vi "Data2Array.vi"(1 "ArrayLen":dbl, 2 "date":dbl) -> (0 "Array":dbl[](array[numeric]))   [LabVIEW 2014, in "Xgraph.xctl"]
uses:
  Xgraph.xctl
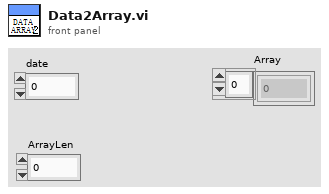
[diagram p1: front panel]
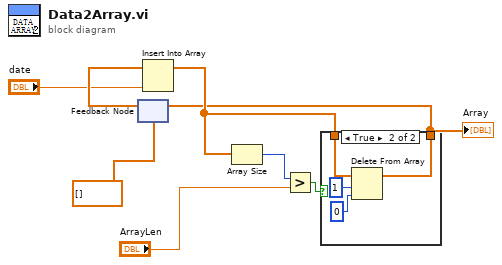
[diagram p0: block diagram]
diagram:
  n1 = feedback #1(dbl[] []) -> (w8:dbl[])
  n2 = Insert Into Array(array=w8, new element="date") -> (w4:dbl[])  [unwired: 1 in]
  n3 = Array Size(array=w4) -> (size(s)=w6:i32)
  n4 = Greater?(x=w6, y="ArrayLen") -> (0:w5:bool)
  n5 = case shown="True" w5 {
    tunnel: w4 -> [w9 w13]
    tunnel: [w9 w12] -> w2
    frame False {
    }
    frame True {
      n6 = Delete From Array(array=w13, length=1, index=0) -> (array with subset deleted=w12:dbl[])  [unwired: 1 out]
    }
  }
  "Array" <- w2
  n7 = feedback-in #1(w2) -> ()
